vi "Load Required Keys.vi"(8 "error in":errorcluster, 9 "Class Path":path, 10 "Cancelled":bool, 11 "Configuration UI in":refnum<class "Configuration UI.lvclass">) -> (0 "error out":errorcluster, 3 "Configuration UI out":refnum<class "Configuration UI.lvclass">)   [LabVIEW 2019, in "Configuration UI.lvlib" / "Configuration UI.lvclass"]
doc: "Open an instance of the instrument type selected to create, call config's <b>Read Required Keys</b> which returns all of the requisite configuration keys and pre-sets the class configuration key to the specific instrument class selected.\n\nThis allows the user to create a well-formed configuration entry in config.ini for the instrument.\n\n<b>***CAUTION***</b>\n\nThe signal list does not currently have this feature, so the instrument class data needs to be inspected to create a well-formed signal list entry for full configuration mapping."
uses:
  Project/Configuration UI.lvclass
  Project/Configuration UI.lvclass/Configuration UI.ctl
  builds/Tools/Config.lvlibp/Config.lvclass
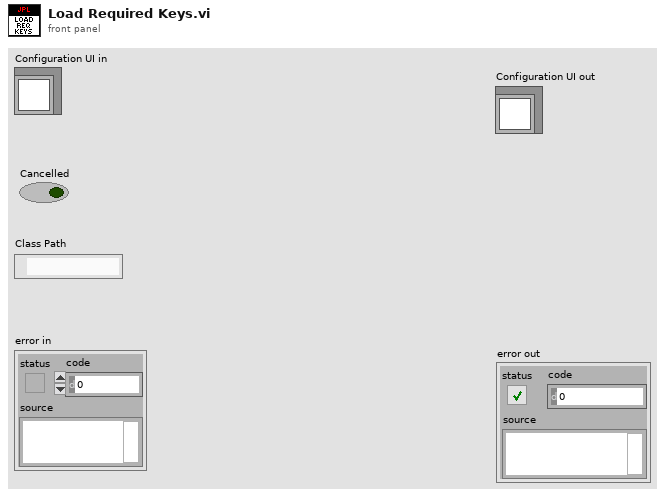
[diagram p1: front panel]
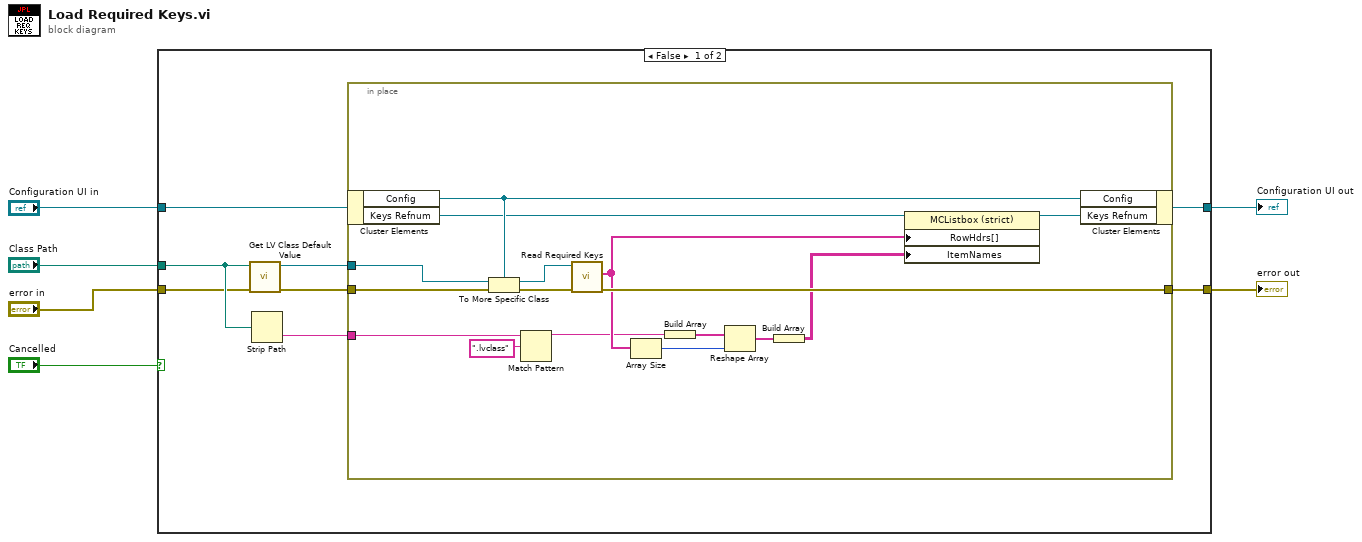
[diagram p0: block diagram]
diagram:
  n1 = case shown="False" "Cancelled" {
    tunnel: "Configuration UI in" -> [w14 w32]
    tunnel: "Class Path" -> [w13 _]
    tunnel: "error in" -> [w12 w31]
    tunnel: [w8 w31] -> w3
    tunnel: [w7 w32] -> w2
    frame False {
      n2 = call <vilib>:"Get LV Class Default Value.vi"("error in (no error)"=w12, "class path"=w13) -> ("error out"=w10:errorcluster, "object"=w11:refnum<class>)  [unwired: 8 in]
      n3 = Strip Path(path=w13) -> (name=w9:string)  [unwired: 1 out]
      n4 = in-place {
        in-place-border: w11 -> [w30]
        in-place-border: w10 -> [w29]
        in-place-border: w9 -> [w26]
        in-place-border: [w24] -> w8
        n5 = in-place-cluster #1(w14) -> ("Config"=w23:refnum<class "Config.lvclass">, "Keys Refnum"=w21:refnum<vi>)
        n6 = To More Specific Class(target class=w23, reference=w30, error in=w29) -> (specific class reference=w28:refnum<class "Config.lvclass">, error out=w27:errorcluster)
        n7 = Match Pattern(string=w26, regular expression=".lvclass") -> (before substring=w19:string)  [unwired: 1 in, 3 out]
        n8 = call "Read Required Keys.vi"("error in (no error)"=w27, "Config in"=w28) -> ("error out"=w24:errorcluster, "Required Keys"=w20:string[])  [unwired: 7 in, 1 out]
        n9 = Array Size(array=w20) -> (size(s)=w17:i32)
        n10 = Build Array(w19) -> (w18:string[])
        n11 = Reshape Array(w18, w17) -> (w16:string[])
        n12 = Build Array(w16) -> (w15:string[][])
        n13 = property class="MCListbox (strict)"(reference=w21, "RowHdrs[]"=w20, "ItemNames"=w15) -> (reference out=w22:refnum<vi>)  [unwired: 1 in, 1 out]
        n14 = in-place-cluster #1("Config"=w23, "Keys Refnum"=w22) -> (w7:refnum<class "Configuration UI.lvclass">)
      }
    }
    frame True {
    }
  }
  "Configuration UI out" <- w2
  "error out" <- w3
